vi "AMAPP Post-Uninstall Custom Action.vi"(10 "Variant":variant) -> (0 "error out":errorcluster)   [LabVIEW 2023]
uses:
  <vilib>/zip/NI_Unzip.lvlib
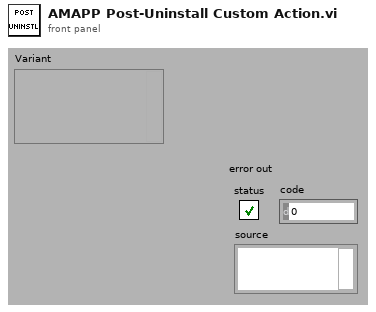
[diagram p1: front panel]
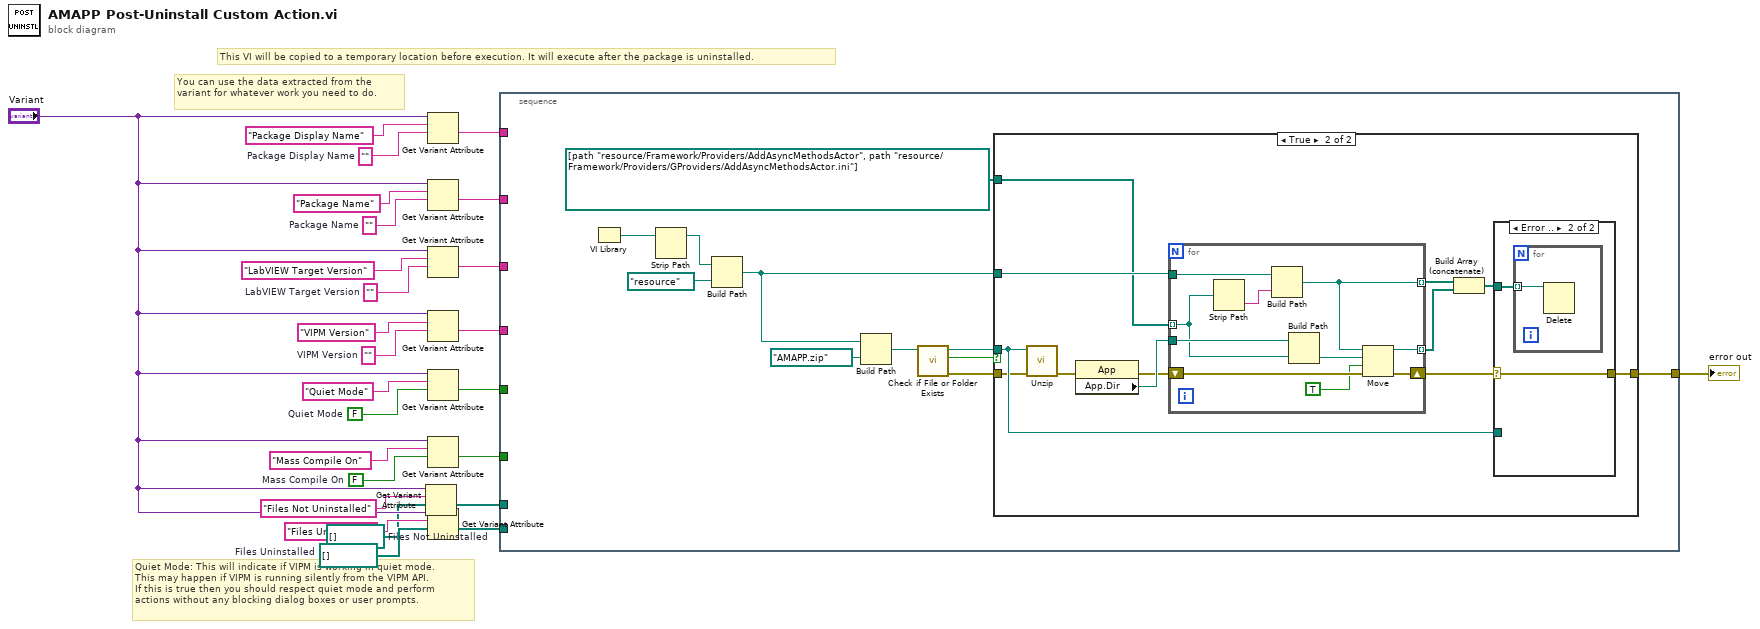
[diagram p0: block diagram]
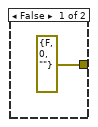
[diagram p2: hidden frame]
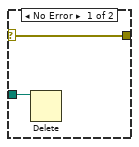
[diagram p3: hidden frame]
diagram:
  w2 = path[] []  # Files Not Uninstalled
  w3 = path[] []  # Files Uninstalled
  w9 = FALSE  # Mass Compile On
  w10 = ""  # Package Display Name
  w17 = FALSE  # Quiet Mode
  w20 = ""  # VIPM Version
  w22 = ""  # LabVIEW Target Version
  w24 = ""  # Package Name
  # "You can use the data extracted from the variant for whatever work you need to do."
  # "Quiet Mode: This will indicate if VIPM is working in quiet mode.\nThis may happen if VIPM is running silently from the VIPM API.\nIf this is true then you should respect quiet mode and perform\nactions without any blocking dialog boxes or user prompts."
  # "This VI will be copied to a temporary location before execution. It will execute after the package is uninstalled."
  n1 = Get Variant Attribute(Variant="Variant", name="Files Not Uninstalled", default value (empty Variant)=w2) -> (value=w7:path[])  [unwired: 1 in, 3 out]
  n2 = Get Variant Attribute(Variant="Variant", name="Package Display Name", default value (empty Variant)=w10) -> (value=w16:string)  [unwired: 1 in, 3 out]
  n3 = Get Variant Attribute(Variant="Variant", name="Package Name", default value (empty Variant)=w24) -> (value=w15:string)  [unwired: 1 in, 3 out]
  n4 = Get Variant Attribute(Variant="Variant", name="LabVIEW Target Version", default value (empty Variant)=w22) -> (value=w14:string)  [unwired: 1 in, 3 out]
  n5 = Get Variant Attribute(Variant="Variant", name="VIPM Version", default value (empty Variant)=w20) -> (value=w13:string)  [unwired: 1 in, 3 out]
  n6 = Get Variant Attribute(Variant="Variant", name="Quiet Mode", default value (empty Variant)=w17) -> (value=w12:bool)  [unwired: 1 in, 3 out]
  n7 = Get Variant Attribute(Variant="Variant", name="Mass Compile On", default value (empty Variant)=w9) -> (value=w11:bool)  [unwired: 1 in, 3 out]
  n8 = Get Variant Attribute(Variant="Variant", name="Files Uninstalled", default value (empty Variant)=w3) -> (value=w6:path[])  [unwired: 1 in, 3 out]
  n9 = stacked-sequence {
    tunnel: w16 -> [_]
    tunnel: w15 -> [_]
    tunnel: w14 -> [_]
    tunnel: w13 -> [_]
    tunnel: w12 -> [_]
    tunnel: w11 -> [_]
    tunnel: w6 -> [_]
    tunnel: w7 -> [_]
    tunnel: [w37] -> w1
    frame #0 {
      n10 = VI Library() -> (path=w35:path)
      n11 = Strip Path(path=w35) -> (stripped path=w33:path)  [unwired: 1 out]
      n12 = Build Path(base path=w33, name or relative path=path "resource") -> (appended path=w32:path)
      n13 = Build Path(base path=w32, name or relative path=path "AMAPP.zip") -> (appended path=w28:path)
      n14 = call <vilib>:"Check if File or Folder Exists.vi"("path"=w28) -> ("error out"=w29:errorcluster, "file or folder exists?"=w30:bool, "dup path"=w27:path)  [unwired: 8 in]
      n15 = case shown="True" w30 {
        tunnel: [errorcluster {"status"=FALSE, "code"=0, "source"=""} ("error IO") w50] -> w37
        tunnel: w32 -> [_ w42]
        tunnel: path[] [path "resource/Framework/Providers/AddAsyncMethodsActor", path "resource/Framework/Providers/GProviders/AddAsyncMethodsActor.ini"] -> [_ w41]
        tunnel: w27 -> [_ w40]
        tunnel: w29 -> [_ w39]
        frame False {
        }
        frame True {
          n16 = call <vilib>:"Unzip.vi"("error in (no error)"=w39, "Zip file"=w40) -> ("error out"=w43:errorcluster)  [unwired: 7 in, 2 out]
          n17 = property class="App"(error in=w43) -> (error out=w44:errorcluster, "App.Dir"=w45:path)  [unwired: 1 in, 1 out]
          n18 = for {
            tunnel: w42 -> [w64]
            shift-right: [w63] -> w49
            shift-left: w44 -> [w65]
            tunnel: w41 -> [w60] mode=indexing
            tunnel: w45 -> [w61]
            tunnel: [w57] -> w46 mode=indexing
            tunnel: [w56] -> w48 mode=indexing
            n19 = Strip Path(path=w60) -> (name=w59:string)  [unwired: 1 out]
            n20 = Build Path(base path=w64, name or relative path=w59) -> (appended path=w57:path)
            n21 = Build Path(base path=w61, name or relative path=w60) -> (appended path=w62:path)
            n22 = Move(source path=w57, error in=w65, 9:TRUE ("overwrite (F)"), 10:w62) -> (error out=w63:errorcluster, 3:w56:path)  [unwired: 1 in, 1 out]
          }
          n23 = Build Array (concatenate)(w46, w48) -> (w47:path[])
          n24 = case shown="Error .." w49 {
            selector: w49 -> [w51 w53]
            tunnel: w47 -> [_ w54]
            tunnel: [w51 w53] -> w50
            tunnel: w40 -> [w52 _]
            frame No Error {
              n25 = Delete(path (use dialog)=w52) -> ()  [unwired: 4 in, 3 out]
            }
            frame Error {
              n26 = for {
                tunnel: w54 -> [w55] mode=indexing
                n27 = Delete(path (use dialog)=w55) -> ()  [unwired: 4 in, 3 out]
              }
            }
          }
        }
      }
    }
  }
  "error out" <- w1
